vi "DuALEX_RN.vi"() -> ()   [LabVIEW 2011]
uses:
  <vilib>/DAQmx/create/channels.llb/DAQmx Create Channel (CO-Pulse Generation-Frequency).vi
  <vilib>/DAQmx/configure/events/hardwareSignals.llb/DAQmx Export Signal (Most Signals).vi
  <vilib>/DAQmx/configure/timing.llb/DAQmx Timing (Implicit).vi
  <vilib>/DAQmx/configure/trigger.llb/DAQmx Start Trigger (Digital Edge).vi
panel:
  in  "Analog Amplitude":dbl=1.0 format="%0.2p"
  in  "Repetition Frequency":dbl=1.0 format="%.6f"
  in  "Stop Button":bool
  # "The  below control is not connected"
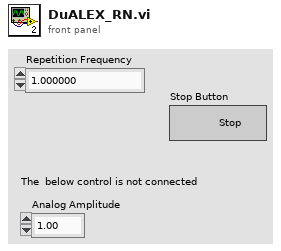
[diagram p1: front panel]
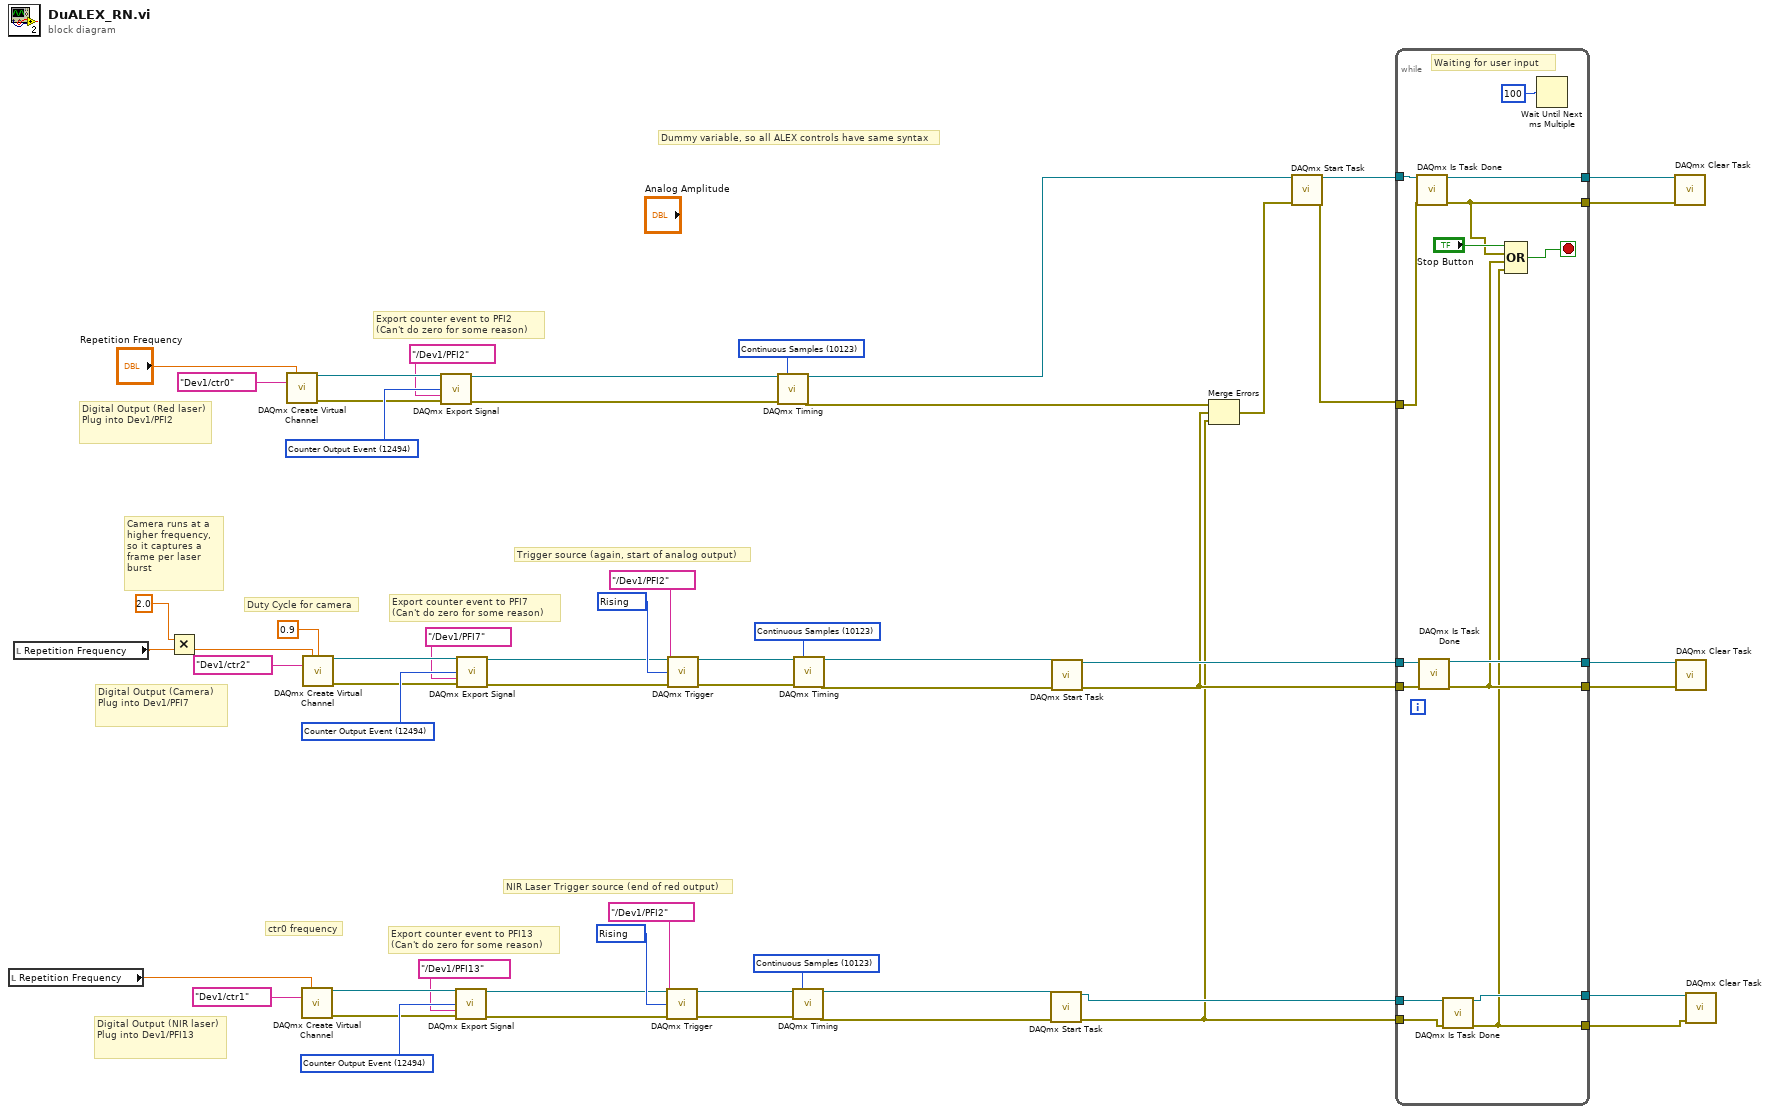
[diagram p0: block diagram]
diagram:
  w17 = 10280 items=["Rising"=10280, "Falling"=10171] ("edge")
  w20 = 10123 items=["Finite Samples"=10178, "Continuous Samples"=10123, "Hardware Timed Single Point"=12522] ("sample mode")
  w22 = 12494 items=["AI Convert Clock"=12484, "10MHz Reference Clock"=12536, "20MHz Timebase Clock"=12486, "Sample Clock"=12487, "Advance Trigger"=12488, "Reference Trigger"=12490, "Start Trigger"=12491, "Advance Complete Event"=12492, "AI Hold Complete Event"=12493, "Counter Output Event"=12494, "Change Detection Event"=12511, "Watchdog Timer Expired Event"=12512] ("signal")
  w39 = 10280 items=["Rising"=10280, "Falling"=10171] ("edge")
  w42 = 10123 items=["Finite Samples"=10178, "Continuous Samples"=10123, "Hardware Timed Single Point"=12522] ("sample mode")
  w44 = 12494 items=["AI Convert Clock"=12484, "10MHz Reference Clock"=12536, "20MHz Timebase Clock"=12486, "Sample Clock"=12487, "Advance Trigger"=12488, "Reference Trigger"=12490, "Start Trigger"=12491, "Advance Complete Event"=12492, "AI Hold Complete Event"=12493, "Counter Output Event"=12494, "Change Detection Event"=12511, "Watchdog Timer Expired Event"=12512] ("signal")
  w54 = 10123 items=["Finite Samples"=10178, "Continuous Samples"=10123, "Hardware Timed Single Point"=12522] ("sample mode")
  w56 = 12494 items=["AI Convert Clock"=12484, "10MHz Reference Clock"=12536, "20MHz Timebase Clock"=12486, "Sample Clock"=12487, "Advance Trigger"=12488, "Reference Trigger"=12490, "Start Trigger"=12491, "Advance Complete Event"=12492, "AI Hold Complete Event"=12493, "Counter Output Event"=12494, "Change Detection Event"=12511, "Watchdog Timer Expired Event"=12512] ("signal")
  # "Dummy variable, so all ALEX controls have same syntax"
  # "Digital Output (NIR laser) Plug into Dev1/PFI13"
  # "NIR Laser Trigger source (end of red output)"
  # "Export counter event to PFI13\n(Can't do zero for some reason)"
  # "ctr0 frequency"
  # "Duty Cycle for camera"
  # "Camera runs at a higher frequency, so it captures a frame per laser burst"
  # "Digital Output (Camera) Plug into Dev1/PFI7"
  # "Trigger source (again, start of analog output)"
  # "Export counter event to PFI7\n(Can't do zero for some reason)"
  # "Digital Output (Red laser) Plug into Dev1/PFI2"
  # "Export counter event to PFI2\n(Can't do zero for some reason)"
  n1 = local read "Repetition Frequency"() -> (w9:dbl)
  n2 = local read "Repetition Frequency"() -> (w31:dbl)
  n3 = Multiply(x=2.0 ("Repetition Frequency"), y=w31) -> (x*y=w30:dbl)
  n4 = call-poly <vilib>:"DAQmx Create Virtual Channel.vi"("frequency"="Repetition Frequency", "counter"=tag "Dev1/ctr0") -> ("task out"=w57:refnum<k21>, "error out"=w55:errorcluster)  [unwired: 12 in]
  n5 = call-poly <vilib>:"DAQmx Create Virtual Channel.vi"("frequency"=w9, "counter"=tag "Dev1/ctr1") -> ("task out"=w23:refnum<k21>, "error out"=w21:errorcluster)  [unwired: 12 in]
  n6 = call-poly <vilib>:"DAQmx Create Virtual Channel.vi"("frequency"=w30, "duty cycle"=0.9, "counter"=tag "Dev1/ctr2") -> ("task out"=w45:refnum<k21>, "error out"=w43:errorcluster)  [unwired: 11 in]
  n7 = call-poly <vilib>:"DAQmx Export Signal.vi"("task/channels in"=w57, "signal"=w56, "output terminal"=tag "/Dev1/PFI2", "error in"=w55) -> ("task out"=w4:refnum<k21>, "error out"=w3:errorcluster)  [unwired: 10 in]
  n8 = call-poly <vilib>:"DAQmx Export Signal.vi"("task/channels in"=w23, "signal"=w22, "output terminal"=tag "/Dev1/PFI13", "error in"=w21) -> ("task out"=w16:refnum<k21>, "error out"=w13:errorcluster)  [unwired: 10 in]
  n9 = call-poly <vilib>:"DAQmx Export Signal.vi"("task/channels in"=w45, "signal"=w44, "output terminal"=tag "/Dev1/PFI7", "error in"=w43) -> ("task out"=w38:refnum<k21>, "error out"=w35:errorcluster)  [unwired: 10 in]
  n10 = call-poly <vilib>:"DAQmx Trigger.vi"("task/channels in"=w16, "source"=tag "/Dev1/PFI2", "edge"=w17, "error in"=w13) -> ("task out"=w15:refnum<k21>, "error out"=w14:errorcluster)  [unwired: 10 in]
  n11 = call-poly <vilib>:"DAQmx Trigger.vi"("task/channels in"=w38, "source"=tag "/Dev1/PFI2", "edge"=w39, "error in"=w35) -> ("task out"=w37:refnum<k21>, "error out"=w36:errorcluster)  [unwired: 10 in]
  n12 = call-poly <vilib>:"DAQmx Timing.vi"("task/channels in"=w4, "sample mode"=w54, "error in"=w3) -> ("task out"=w2:refnum<k21>, "error out"=w1:errorcluster)  [unwired: 11 in]
  n13 = call-poly <vilib>:"DAQmx Timing.vi"("task/channels in"=w15, "sample mode"=w20, "error in"=w14) -> ("task out"=w12:refnum<k21>, "error out"=w11:errorcluster)  [unwired: 11 in]
  n14 = call-poly <vilib>:"DAQmx Timing.vi"("task/channels in"=w37, "sample mode"=w42, "error in"=w36) -> ("task out"=w34:refnum<k21>, "error out"=w33:errorcluster)  [unwired: 11 in]
  n15 = call <vilib>:"DAQmx Start Task.vi"("task/channels in"=w12, "error in"=w11) -> ("task out"=w8:refnum<k21>, "error out"=w7:errorcluster)  [unwired: 12 in]
  n16 = call <vilib>:"DAQmx Start Task.vi"("task/channels in"=w34, "error in"=w33) -> ("task out"=w27:refnum<k21>, "error out"=w26:errorcluster)  [unwired: 12 in]
  n17 = Merge Errors(w1, w26, w7) -> (w52:errorcluster)
  n18 = call <vilib>:"DAQmx Start Task.vi"("task/channels in"=w2, "error in"=w52) -> ("task out"=w51:refnum<k21>, "error out"=w50:errorcluster)  [unwired: 12 in]
  n19 = while {
    tunnel: [w72] -> w48
    tunnel: [w58] -> w49
    tunnel: w51 -> [w69]
    tunnel: w50 -> [w68]
    tunnel: w27 -> [w67]
    tunnel: w26 -> [w66]
    tunnel: [w64] -> w25
    tunnel: [w63] -> w24
    tunnel: w8 -> [w62]
    tunnel: w7 -> [w61]
    tunnel: [w60] -> w6
    tunnel: [w59] -> w5
    stop <- w70 stop-if-true
    # "Waiting for user input"
    n20 = call <vilib>:"DAQmx Is Task Done.vi"("task/channels in"=w69, "error in"=w68) -> ("task out"=w72:refnum<k21>, "error out"=w58:errorcluster)  [unwired: 11 in, 1 out]
    n21 = call <vilib>:"DAQmx Is Task Done.vi"("task/channels in"=w67, "error in"=w66) -> ("task out"=w64:refnum<k21>, "error out"=w63:errorcluster)  [unwired: 11 in, 1 out]
    n22 = call <vilib>:"DAQmx Is Task Done.vi"("task/channels in"=w62, "error in"=w61) -> ("task out"=w60:refnum<k21>, "error out"=w59:errorcluster)  [unwired: 11 in, 1 out]
    n23 = Compound Arithmetic op=OR("Stop Button", w58, w63, w59) -> (w70:bool)
    n24 = Wait Until Next ms Multiple(millisecond multiple=u32 100) -> ()  [unwired: 1 out]
  }
  n25 = call <vilib>:"DAQmx Clear Task.vi"("task in"=w48, "error in"=w49) -> ()  [unwired: 13 in, 1 out]
  n26 = call <vilib>:"DAQmx Clear Task.vi"("task in"=w25, "error in"=w24) -> ()  [unwired: 13 in, 1 out]
  n27 = call <vilib>:"DAQmx Clear Task.vi"("task in"=w6, "error in"=w5) -> ()  [unwired: 13 in, 1 out]
